vi "WLC Fitting_Final_v3_YCC.vi"(3 "initial parameters (Lp,Lc) or (Lc,K)":dbl[](array[numeric])=[40.0, 1750.0], 4 "Fitting Cluster":T1={"cr (um)"=0.0, "yr (V)"=0.0, "trap height(nm)"=300.0, "bead radius(nm)"=515.0, "Length offset"=550.0, "Upper Force(pN)"=500.0, "cr shift (nm)"=0.0, "yr shift (mV)"=0.0, "LaserPower (mW)"=4500.0, "conversion factor (V/um)"=0.0, "Stiffness (pN/nm)"=0.0, "xDNA cut outside"=3000.0, "Lower Force(pN)"=5.0, "c for zbd"=0.002} {"c for zbd" format="%_6g"}, 5 "Enum":T2(ring)=enum."direct fit (Lp,Lc,K)", 6 "Load Stage-QPD data":path, 7 "T=Fit U or twoside\nF=Fit F":bool=TRUE, 8 "F+U data?":bool=TRUE, 9 "Finish Fitting":bool, 10 "Ready to Fit":bool, 11 "DataRecord type":enum32{"OneDirectionOnly?", "TwoSide Data"}(tab)) -> (0 "best fit parameters":dbl[](array[numeric]), 1 "r^2":dbl)   [LabVIEW 2014]
uses:
  SubVI/WLC-Fitting Cluster.ctl
  <vilib>/Utility/file.llb/Read From Spreadsheet File (DBL).vi
  <vilib>/gmath/NumericalOptimization/Nonlinear Curve Fit LM formula string.vi
  <vilib>/Utility/file.llb/Write To Spreadsheet File (DBL).vi
  <vilib>/gmath/NI_Gmath.lvlib
panel:
  out "error out":errorcluster
  in  "Given Lp (nm)":dbl=5.0
  in  "Lower Force (pN)":dbl=6.0
  in  "Upper Force (pN)":dbl=45.0
  in  "Set lower foce offset?":bool
  out "U-Force or twoside 2":dbl[](array[numeric])
  out "U-xDNA or twoside 2":dbl[](array[numeric])
  in  "initial guess K (pN)":dbl=1200.0
  out "OneDirectionOnly?":bool=TRUE
  in  "Fit \"+\"(RHS) ?":bool=TRUE
  in  "Fit One Side?":bool
  in  "Reverse sign?":bool=TRUE
  out "Cut-Force for eWLC (pN)":dbl[](array[numeric])
  out "best nonlinear fit extension (eWLC)":dbl[](array[numeric])
  in  "T=use stuckbead 7th order\nF=use slope 1st order calibrate":bool
  out "Force to be saved":dbl[](array[numeric])
  out "xDNA to be saved":dbl[](array[numeric])
  out "F-Force":dbl[](array[numeric])
  out "F-xDNA":dbl[](array[numeric])
  in  "F-yr shift (mV)":dbl
  in  "F-cr shift (nm)":dbl
  out "F-QPD signal (V)":dbl[](array[numeric])
  out "F-Stage Positions (um)":dbl[](array[numeric])
  in  "stuckbead path (dialog if empty)":path=path "D:/Calibration-Stuckbead-Scan/20181220/2/202224-x-Stuckbead Scan-6000.00-step 5.00 nm-QPD height 3.340-h0.txt"
  out "Save to Path":path
  out "best nonlinear fit force (M-S)":dbl[](array[numeric])
  in  "SaveName":enum16{"ForecExtension Only", "WLC Fitting"}(ring)
  in  "Save Calibrated Data?":bool
  out "U-Force or twoside":dbl[](array[numeric])
  out "U-xDNA or twoside":dbl[](array[numeric])
  out "Fitting Cluster for indicator":T1={"cr (um)"=0.0, "yr (V)"=0.0, "trap height(nm)"=0.0, "bead radius(nm)"=520.0, "Length offset"=0.0, "Upper Force(pN)"=0.0, "cr shift (nm)"=0.0, "yr shift (mV)"=0.0, "LaserPower (mW)"=0.0, "conversion factor (V/um)"=0.0, "Stiffness (pN/nm)"=0.0154, "xDNA cut outside"=0.0, "Lower Force(pN)"=5.0, "c for zbd"=0.0}
  in  "Tab Control":T3(tab)
  out "Stage-QPD Graph":T4(graph)
  out "U-Extension-Force Graph":cluster{"xDNA":dbl[], "Force":dbl[]}(graph)
  out "F-Extension-Force Graph":cluster{"xDNA":dbl[], "Force":dbl[]}(graph)
  out "All-Extension-Force Graph":T5(graph)
  out "Extension-Force and WLC Graph":cluster{"xDNA":dbl[], "Force":dbl[]}[](graph)
  out "All Extension-Force and WLC Graph":T6(graph)
  in  "Delete Outside Signal?":bool
  out "U-QPD signal or All QPD  (V)":dbl[](array[numeric])
  out "U-Stage Positions or All stage positions (um)":dbl[](array[numeric])
  out "Read-Extension (nm)":dbl[](array[numeric])
  out "Read-Force (pN)":dbl[](array[numeric])
  in  "T=Read QPD-Stage data\nF=Read Force-Extension data":bool=TRUE
  # "5180bp=1750.8 nm\n3281bp=1109.0 nm"
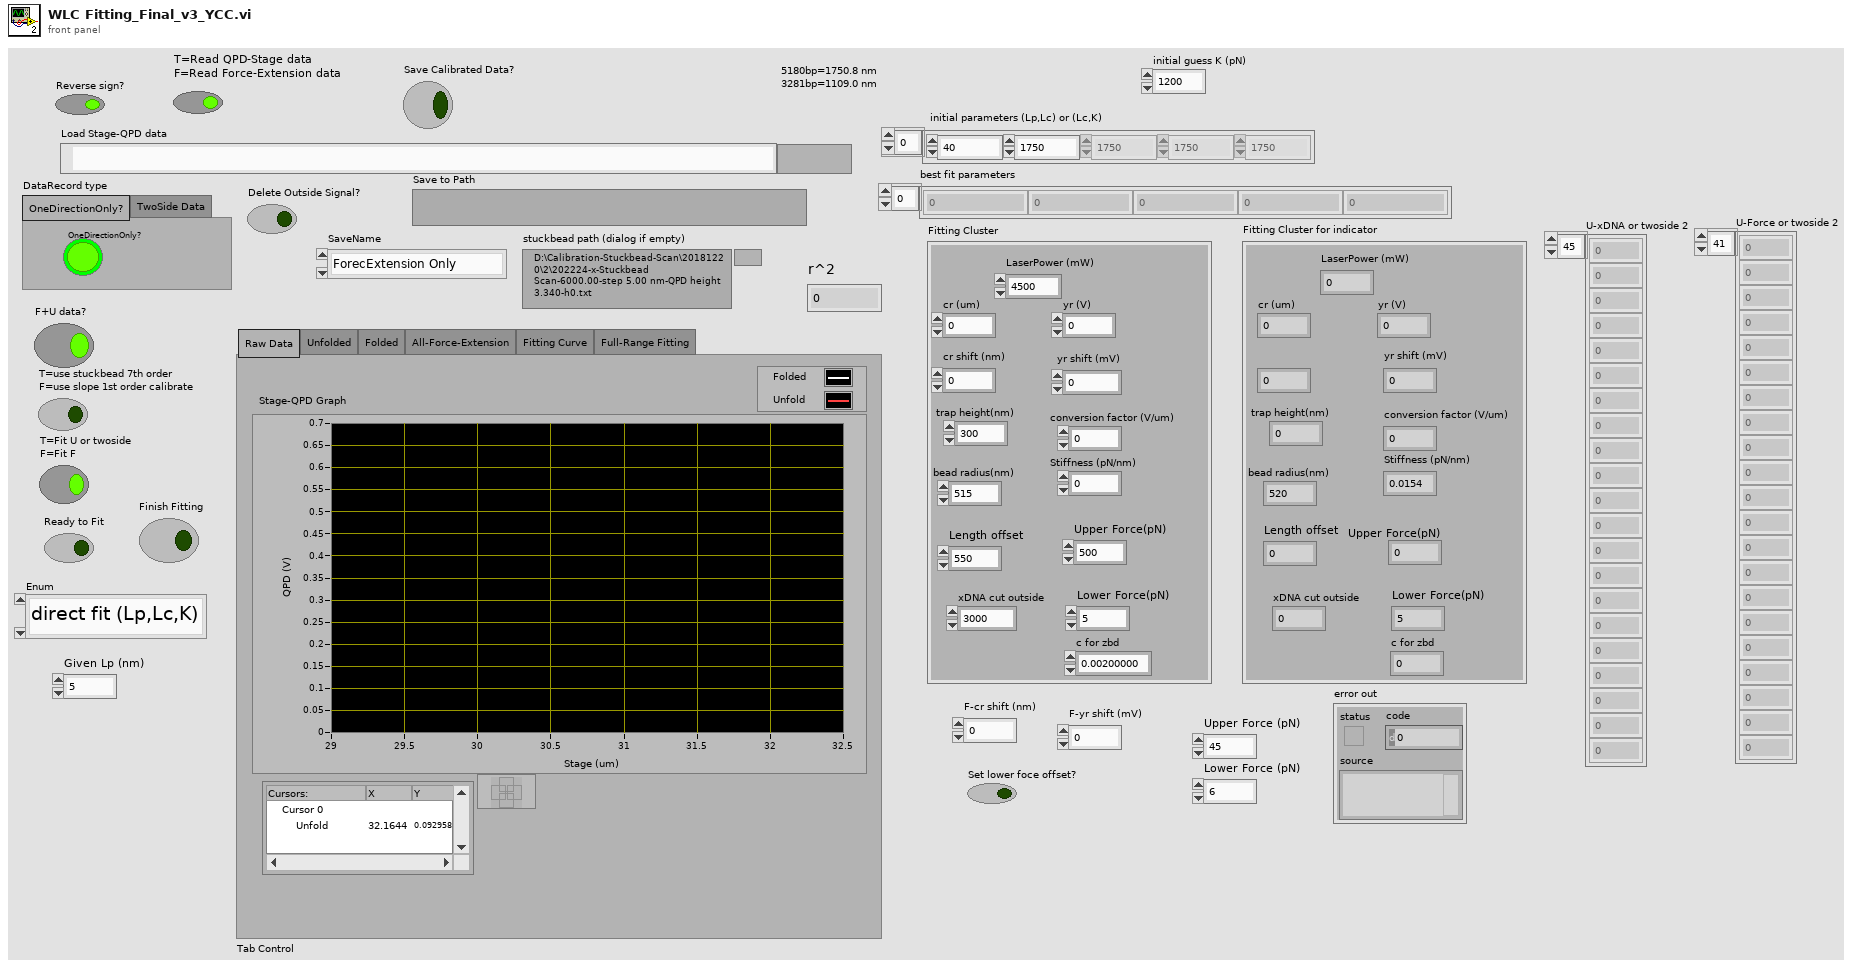
[diagram p1: front panel]
types:
  T1 = typedef "WLC-Fitting Cluster.ctl" = cluster{"cr (um)":dbl, "yr (V)":dbl, "trap height(nm)":dbl, "bead radius(nm)":dbl, "Length offset":dbl, "Upper Force(pN)":dbl, "cr shift (nm)":dbl, "yr shift (mV)":dbl, "LaserPower (mW)":dbl, "conversion factor (V/um)":dbl, "Stiffness (pN/nm)":dbl, "xDNA cut outside":dbl, "Lower Force(pN)":dbl, "c for zbd":dbl}
  T2 = enum16{" Marko-Siggia for centering", "Marko-Siggia", "direct fit (Lp,Lc,K)", "fit K (Lp,Lc,K)", "eWLC (Lp=45,Lc,K)"}
  T3 = enum32{"Raw Data", "Unfolded", "Folded", "All-Force-Extension", "Fitting Curve", "Full-Range Fitting"}
  T4 = cluster{"Sorted Stage Position (um)":dbl[], "Sorted QPD (V)":dbl[]}[]
  T5 = cluster{"Folded-xDNA":dbl[], "Folded-Force":dbl[]}[]
  T6 = cluster{"cut-full xDNA":dbl[], "cut-full Force":dbl[]}[]
  T7 = cluster{"model":string, "Parameters":string[], "x":string}
  T8 = cluster{"F-Stage Positions (um) ":dbl[], "F-QPD signal (V) ":dbl[]}
  T9 = cluster{"U-Stage Positions or All stage positions (um)":dbl[], "U-QPD signal or All QPD  (V)":dbl[]}
  T10 = cluster{"U-Stage Positions or All stage positions (um)":dbl[], "U-QPD signal or All QPD  (V)":dbl[]}[]
  T11 = cluster{"Folded-xDNA":dbl[], "Folded-xDNA":dbl[]}
  T12 = cluster{"cut-full xDNA":dbl[], "best nonlinear fit":dbl[]}
  T13 = cluster{"best nonlinear fit":dbl[], "cut-full Force":dbl[]}
  T14 = cluster{"cut-full xDNA":dbl[], "cut-full Force":dbl[]}
  T15 = cluster{"Fit Extension (nm)":dbl[], "Fit Force (pN)":dbl[]}
  T16 = cluster{"xDNA to be saved":dbl[], "Force to be saved":dbl[]}
  T17 = cluster{"xDNA to be saved":dbl[], "Force to be saved":dbl[]}[]
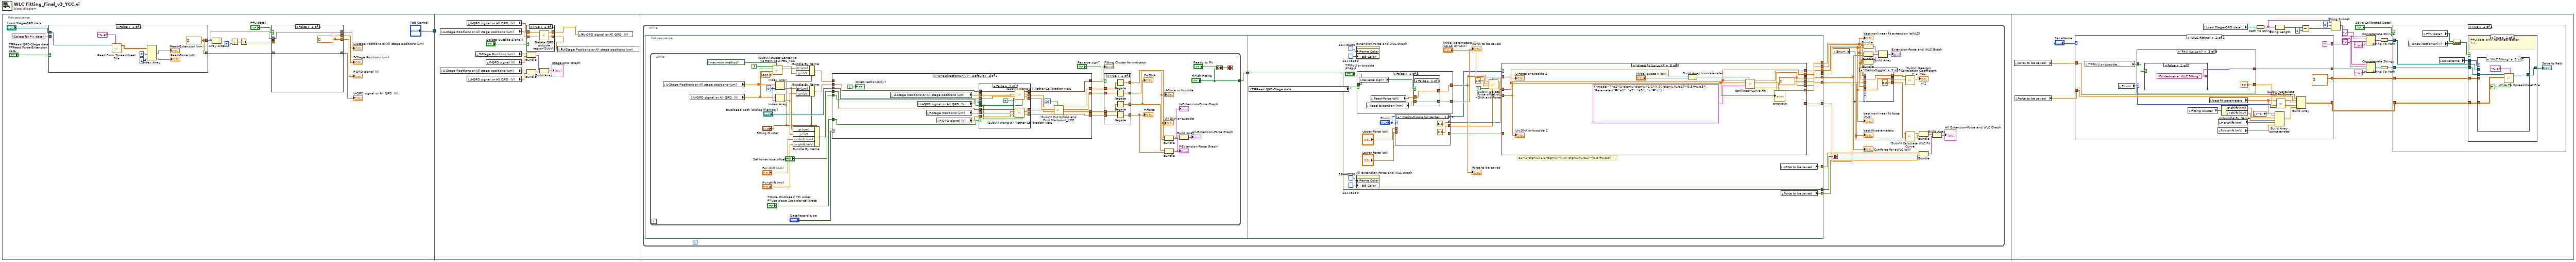
[diagram p0: block diagram]
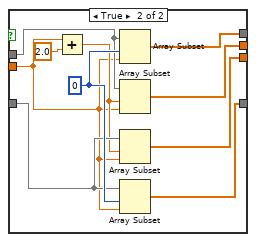
[diagram p2: hidden frame]
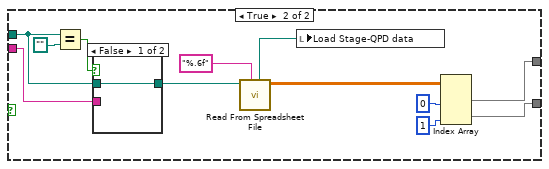
[diagram p3: hidden frame]
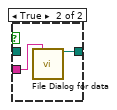
[diagram p4: hidden frame]
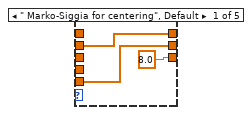
[diagram p6: hidden frame]
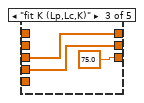
[diagram p7: hidden frame]
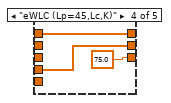
[diagram p8: hidden frame]
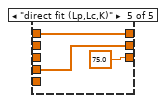
[diagram p9: hidden frame]
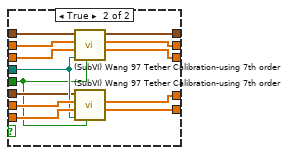
[diagram p11: hidden frame]
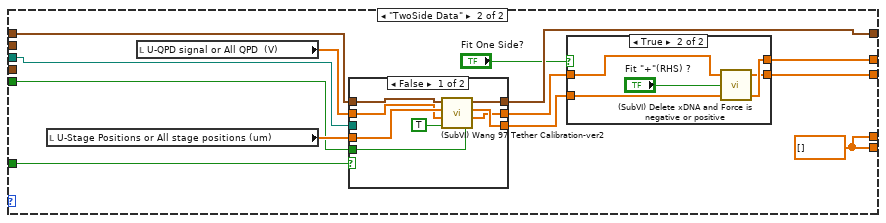
[diagram p12: hidden frame]
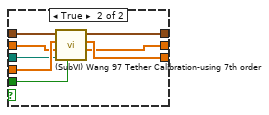
[diagram p14: hidden frame]
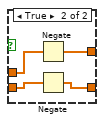
[diagram p15: hidden frame]
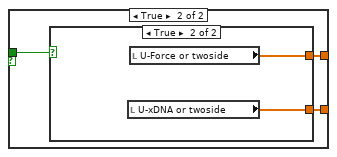
[diagram p16: hidden frame]
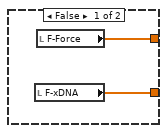
[diagram p17: hidden frame]
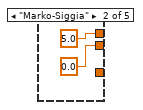
[diagram p18: hidden frame]
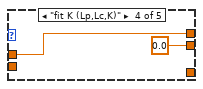
[diagram p20: hidden frame]
diagram:
  n1 = flat-sequence {
    tunnel: ["Tab Control"] -> w1
    tunnel: w1 -> [_]
    frame #0 {
      n2 = case shown="False" "T=Read QPD-Stage data\nF=Read Force-Extension data" {
        tunnel: [w35 w45] -> w11
        tunnel: [w35 w46] -> w6
        tunnel: "Select for F-x data" ("default name") -> [_ w42]
        tunnel: "Load Stage-QPD data" -> [w37 w39]
        frame False {
          w35 = dbl[] [] ("all rows")
          n3 = call-poly <vilib>:"Read From Spreadsheet File.vi"("format (%.3f)"="%.6f", "file path (dialog if empty)"=w37) -> ("all rows"=w32:dbl[][])  [unwired: 5 in, 4 out]
          n4 = Index Array(array=w32, index (col) #1=0 ("disabled index (col)"), index (col) #2=1 ("index (col)")) -> (element #1=→"Read-Extension (nm)":dbl[], element #2=→"Read-Force (pN)":dbl[])  [unwired: 2 in]
        }
        frame True {
          n5 = Equal?(x=w39, y=path "") -> (x = y?=w40:bool)
          n6 = case shown="False" w40 {
            tunnel: [w50 w51] -> w43
            tunnel: w42 -> [_ w52]
            tunnel: w39 -> [w50 _]
            frame False {
            }
            frame True {
              n7 = call "File Dialog for data"("prompt"=w52) -> ("selected path"=w51:path)  [unwired: 11 in, 3 out]
            }
          }
          n8 = call-poly <vilib>:"Read From Spreadsheet File.vi"("format (%.3f)"="%.6f", "file path (dialog if empty)"=w43) -> ("all rows"=w49:dbl[][], "new file path (Not A Path if cancelled)"=w38:path)  [unwired: 5 in, 3 out]
          n9 = local write "Load Stage-QPD data"(w38) -> ()
          n10 = Index Array(array=w49, index (col) #1=0 ("disabled index (col)"), index (col) #2=1 ("index (col)")) -> (element #1=w46:dbl[], element #2=w45:dbl[])  [unwired: 2 in]
        }
      }
      n11 = Array Size(array=w6) -> (size(s)=w7:i32)
      n12 = Divide(x=w7, y=2) -> (x/y=w5:dbl)
      n13 = Decrement(x=w5) -> (x-1=w4:dbl)
      n14 = case shown="False" "F+U data?" {
        tunnel: w6 -> [w19 w25]
        tunnel: w11 -> [w18 w26]
        tunnel: [w19 w29] -> w10
        tunnel: [w18 w27] -> w9
        tunnel: w4 -> [_ w20]
        tunnel: [w17 w24] -> w3
        tunnel: [w17 w23] -> w2
        frame False {
          w17 = dbl[] []
        }
        frame True {
          w28 = 0 ("index")
          n15 = Add(x=w20, y=2.0) -> (x+y=w21:dbl)
          n16 = Array Subset(array=w25, index=w28, length=w20) -> (w29:dbl[])
          n17 = Array Subset(array=w25, index=w21, length=w20) -> (w24:dbl[])
          n18 = Array Subset(array=w26, index=w21, length=w20) -> (w23:dbl[])
          n19 = Array Subset(array=w26, index=w28, length=w20) -> (w27:dbl[])
        }
      }
      "U-Stage Positions or All stage positions (um)" <- w10
      "U-QPD signal or All QPD  (V)" <- w9
      "F-Stage Positions (um)" <- w3
      "F-QPD signal (V)" <- w2
    }
    frame #1 {
      n20 = local read "U-Stage Positions or All stage positions (um)"() -> (w63:dbl[])
      n21 = local read "U-Stage Positions or All stage positions (um)"() -> (w61:dbl[])
      n22 = local read "U-QPD signal or All QPD  (V)"() -> (w62:dbl[])
      n23 = local read "U-QPD signal or All QPD  (V)"() -> (w60:dbl[])
      n24 = local read "F-Stage Positions (um)"() -> (w56:dbl[])
      n25 = local read "F-QPD signal (V)"() -> (w55:dbl[])
      n26 = case shown="True" "Delete Outside Signal?" {
        tunnel: w62 -> [w66 w70]
        tunnel: w63 -> [w65 w69]
        tunnel: [w66 w68] -> w53
        tunnel: [w65 w67] -> w54
        frame False {
        }
        frame True {
          n27 = call "Delete QPD outside region(SubVI).vi"("Position Array In"=w69, "QPD signal In"=w70) -> ("Position Array Out"=w67:dbl[], "QPD signal Out"=w68:dbl[])  [unwired: 8 in]
        }
      }
      n28 = Bundle("F-Stage Positions (um)"=w56, "F-QPD signal (V)"=w55) -> (w59:T8)  [unwired: 1 in]
      n29 = Bundle("U-Stage Positions or All stage positions (um)"=w61, "U-QPD signal or All QPD  (V)"=w60) -> (w58:T9)  [unwired: 1 in]
      n30 = Build Array(w59, w58) -> (→"Stage-QPD Graph":T10)
      n31 = local write "U-Stage Positions or All stage positions (um)"(w54) -> ()
      n32 = local write "U-QPD signal or All QPD  (V)"(w53) -> ()
    }
    frame #2 {
      n33 = while {
        stop <- w85 stop-if-true
        n34 = flat-sequence {
          tunnel: [w111] -> w86
          tunnel: [w269] -> w91
          tunnel: [w268] -> w82
          tunnel: [w266] -> w88
          tunnel: [w265] -> w92
          tunnel: [w264] -> w87
          tunnel: [w263] -> w94
          tunnel: [w262] -> w85
          tunnel: w86 -> [w262]
          tunnel: [w249] -> w83
          tunnel: [w248] -> w74
          tunnel: [w247] -> w73
          frame #0 {
            n35 = while {
              tunnel: ["Finish Fitting"] -> w111
              stop <- w115 stop-if-true
              w147 = 0 ("index")
              n36 = local read "U-Stage Positions or All stage positions (um)"() -> (w136:dbl[])
              n37 = local read "U-QPD signal or All QPD  (V)"() -> (w135:dbl[])
              n38 = call "(SubVI) Guess Center xc yc From Raw FEC_YCC.vi"("Enum"=enum16{"parity method", "max-min method"}."max-min method", "avg range for QPD center (nm)"=600.0, "QPD array (V)"=w135, "Stage array(um)"=w136, "Read data?"=FALSE) -> ("Guess-QPD-center (V)"=w133:dbl, "Guess-stage-center(um)"=w134:dbl)  [unwired: 1 in, 2 out]
              n39 = Index Array(array=w136, index=w147) -> (element=w144:dbl)
              n40 = Index Array(array=w135, index=w147) -> (element=w143:dbl)
              n41 = Bundle By Name(cluster="Fitting Cluster", "cr (um)"=w144, "yr (V)"=w143, "cr shift (nm)"="F-cr shift (nm)", "yr shift (mV)"="F-yr shift (mV)") -> (w140:T1)
              n42 = Bundle By Name(cluster="Fitting Cluster", "cr (um)"=w134, "yr (V)"=w133) -> (w132:T1)
              n43 = Bundle By Name(cluster="Fitting Cluster", "cr (um)"=w144, "yr (V)"=w143) -> (w146:T1)
              n44 = case shown="\"OneDirectionOnly?\", Default" "DataRecord type" {
                tunnel: w146 -> [w177 _]
                tunnel: [w178 w215] -> w145
                tunnel: w140 -> [w173 _]
                tunnel: w132 -> [_ w218]
                tunnel: [w167 w208] -> w129
                tunnel: [w166 w207] -> w123
                tunnel: [w165 w214] -> w128
                tunnel: [w164 w214] -> w127
                tunnel: "T=use stuckbead 7th order\nF=use slope 1st order calibrate" -> [w163 w213]
                tunnel: "stuckbead path (dialog if empty)" -> [w162 w212]
                tunnel: "Set lower foce offset?" -> [w160 w206]
                frame "OneDirectionOnly?", Default {
                  n45 = local read "U-Stage Positions or All stage positions (um)"() -> (w176:dbl[])
                  n46 = local read "U-QPD signal or All QPD  (V)"() -> (w179:dbl[])
                  n47 = local read "F-Stage Positions (um)"() -> (w175:dbl[])
                  n48 = local read "F-QPD signal (V)"() -> (w174:dbl[])
                  n49 = case shown="False" w163 {
                    tunnel: w179 -> [w191 w205]
                    tunnel: [w190 w204] -> w178
                    tunnel: w177 -> [w182 w203]
                    tunnel: w176 -> [w192 w202]
                    tunnel: w175 -> [w188 w201]
                    tunnel: w174 -> [w187 w200]
                    tunnel: w162 -> [_ w199]
                    tunnel: w173 -> [w189 w198]
                    tunnel: [w186 w197] -> w171
                    tunnel: [w185 w196] -> w170
                    tunnel: [w184 w195] -> w169
                    tunnel: [w183 w194] -> w168
                    tunnel: w160 -> [w180 w193]
                    frame False {
                      w181 = TRUE ("X=T\nY=F")
                      n50 = call "(SubVI) Wang 97 Tether Calibration-ver2.vi"("Set lower foce offset?"=w180, "X=T\nY=F"=w181, "QPD signal"=w191, "Stage Position"=w192, "Fitting Cluster"=w182) -> ("Force"=w185:dbl[], "xDNA"=w186:dbl[], "output cluster"=w190:T1)
                      n51 = call "(SubVI) Wang 97 Tether Calibration-ver2.vi"("Set lower foce offset?"=w180, "X=T\nY=F"=w181, "QPD signal"=w187, "Stage Position"=w188, "Fitting Cluster"=w189) -> ("Force"=w183:dbl[], "xDNA"=w184:dbl[])  [unwired: 1 out]
                    }
                    frame True {
                      n52 = call "(SubVI) Wang 97 Tether Calibration-using 7th order.vi"("Set lower foce offset?"=w193, "stuckbead path (dialog if empty)"=w199, "QPD signal"=w205, "Stage Position"=w202, "Fitting Cluster"=w203) -> ("Force"=w196:dbl[], "xDNA"=w197:dbl[], "output cluster"=w204:T1)  [unwired: 2 in, 2 out]
                      n53 = call "(SubVI) Wang 97 Tether Calibration-using 7th order.vi"("Set lower foce offset?"=w193, "stuckbead path (dialog if empty)"=w199, "QPD signal"=w200, "Stage Position"=w201, "Fitting Cluster"=w198) -> ("Force"=w194:dbl[], "xDNA"=w195:dbl[])  [unwired: 2 in, 3 out]
                    }
                  }
                  n54 = call "(SubVI) Cut Unfold and Fold Startpoint_YCC.vi"("number to cut"=10, "Folded-Force in"=w168, "Folded-xDNA in"=w169, "Unfolded-Force"=w170, "Unfolded-xDNA"=w171) -> ("Folded-Force"=w164:dbl[], "Folded-xDNA"=w165:dbl[], "Unfolded-Force"=w166:dbl[], "Unfolded-xDNA"=w167:dbl[])  [unwired: 3 in]
                  "OneDirectionOnly?" <- TRUE
                }
                frame "TwoSide Data" {
                  w214 = dbl[] [] ("Folded-xDNA")
                  n55 = local read "U-Stage Positions or All stage positions (um)"() -> (w217:dbl[])
                  n56 = local read "U-QPD signal or All QPD  (V)"() -> (w216:dbl[])
                  n57 = case shown="False" w213 {
                    tunnel: w218 -> [w233 w241]
                    tunnel: w217 -> [w232 w240]
                    tunnel: w216 -> [w231 w239]
                    tunnel: [w230 w237] -> w215
                    tunnel: [w229 w236] -> w209
                    tunnel: [w228 w235] -> w210
                    tunnel: w212 -> [_ w238]
                    tunnel: w206 -> [w226 w234]
                    frame False {
                      n58 = call "(SubVI) Wang 97 Tether Calibration-ver2.vi"("Set lower foce offset?"=w226, "X=T\nY=F"=TRUE ("X=T\nY=F"), "QPD signal"=w231, "Stage Position"=w232, "Fitting Cluster"=w233) -> ("Force"=w228:dbl[], "xDNA"=w229:dbl[], "output cluster"=w230:T1)
                    }
                    frame True {
                      n59 = call "(SubVI) Wang 97 Tether Calibration-using 7th order.vi"("Set lower foce offset?"=w234, "stuckbead path (dialog if empty)"=w238, "QPD signal"=w239, "Stage Position"=w240, "Fitting Cluster"=w241) -> ("Force"=w235:dbl[], "xDNA"=w236:dbl[], "output cluster"=w237:T1)  [unwired: 2 in, 2 out]
                    }
                  }
                  n60 = case shown="True" "Fit One Side?" {
                    tunnel: w210 -> [w220 w224]
                    tunnel: w209 -> [w219 w223]
                    tunnel: [w219 w222] -> w208
                    tunnel: [w220 w221] -> w207
                    frame False {
                    }
                    frame True {
                      n61 = call "(SubVI) Delete xDNA and Force is negative or positive.vi"("xDNA"=w223, "T=positive (RHS)\nF=negative (LHS)"="Fit \"+\"(RHS) ?", "Force"=w224) -> ("xDNA-cut"=w222:dbl[], "Force-cut"=w221:dbl[])  [unwired: 1 in]
                    }
                  }
                }
              }
              "Fitting Cluster for indicator" <- w145
              n62 = case shown="True" "Reverse sign?" {
                tunnel: w129 -> [w151 w153]
                tunnel: w128 -> [w149 w159]
                tunnel: w127 -> [w148 w158]
                tunnel: [w148 w157] -> w126
                tunnel: [w149 w156] -> w125
                tunnel: [w151 w152] -> w124
                tunnel: w123 -> [w150 w155]
                tunnel: [w150 w154] -> w122
                frame False {
                }
                frame True {
                  n63 = Negate(x=w153) -> (-x=w152:dbl[])
                  n64 = Negate(x=w155) -> (-x=w154:dbl[])
                  n65 = Negate(x=w159) -> (-x=w156:dbl[])
                  n66 = Negate(x=w158) -> (-x=w157:dbl[])
                }
              }
              "U-xDNA or twoside" <- w124
              "U-Force or twoside" <- w122
              "F-xDNA" <- w125
              "F-Force" <- w126
              n67 = Bundle("xDNA-cut"=w124, "Force-cut"=w122) -> (w137:cluster{"xDNA-cut":dbl[], "Force-cut":dbl[]})  [unwired: 1 in]
              "U-Extension-Force Graph" <- w137
              n68 = Bundle("Folded-xDNA"=w125, "Folded-xDNA"=w126) -> (w138:T11)  [unwired: 1 in]
              "F-Extension-Force Graph" <- w138
              n69 = Build Array(w138, w137) -> (→"All-Extension-Force Graph":cluster{"xDNA-cut":dbl[], "Force-cut":dbl[]}[])
              n70 = Or(x="Ready to Fit", y="Finish Fitting") -> (x .or. y?=w115:bool)
            }
          }
          frame #1 {
            # "a2*(1*sign(u)-1/2*sign(u)*(4.07/sign(u)/u/a1)**(0.5)+u/a3);"
            n71 = local read "T=Read QPD-Stage data\nF=Read Force-Extension data"() -> (w242:bool)
            n72 = property on="Extension-Force and WLC Graph" class="XYGraph (strict)"("Frame Color"=u32 16448250, "BG Color"=u32 16448250) -> ()  [unwired: 2 in, 2 out]
            n73 = property on="All Extension-Force and WLC Graph" class="XYGraph (strict)"("Frame Color"=u32 16448250, "BG Color"=u32 16448250) -> ()  [unwired: 2 in, 2 out]
            n74 = case shown="False" w242 {
              tunnel: "T=Fit U or twoside\nF=Fit F" -> [_ w284]
              tunnel: [w271 w283] -> w257
              tunnel: [w272 w282] -> w256
              frame False {
                n75 = local read "Reverse sign?"() -> (w275:bool)
                n76 = local read "Read-Extension (nm)"() -> (w273:dbl[])
                n77 = local read "Read-Force (pN)"() -> (w274:dbl[])
                n78 = case shown="False" w275 {
                  tunnel: w274 -> [w277 w281]
                  tunnel: w273 -> [w276 w279]
                  tunnel: [w277 w280] -> w272
                  tunnel: [w276 w278] -> w271
                  frame False {
                  }
                  frame True {
                    n79 = Negate(x=w281) -> (-x=w280:dbl[])
                    n80 = Negate(x=w279) -> (-x=w278:dbl[])
                  }
                }
              }
              frame True {
                n81 = case shown="True" w284 {
                  tunnel: [w286 w288] -> w283
                  tunnel: [w285 w287] -> w282
                  frame False {
                    n82 = local read "F-xDNA"() -> (w286:dbl[])
                    n83 = local read "F-Force"() -> (w285:dbl[])
                  }
                  frame True {
                    n84 = local read "U-xDNA or twoside"() -> (w288:dbl[])
                    n85 = local read "U-Force or twoside"() -> (w287:dbl[])
                  }
                }
              }
            }
            "xDNA to be saved" <- w257
            "Force to be saved" <- w256
            n86 = case shown="\" Marko-Siggia for centering\", Default" "Enum" {
              tunnel: [0.0 0.0 w293 0.0 ("Lower Force (pN)") w298] -> w254
              tunnel: [5.0 5.0 w294 w295 w299] -> w253
              tunnel: "Upper Force (pN)" -> [_ _ w294 w295 w299]
              tunnel: "Lower Force (pN)" -> [_ _ w293 _ w298]
              tunnel: [_ _ _ _ "Given Lp (nm)"] -> w250
              frame " Marko-Siggia for centering", Default {
              }
              frame "Marko-Siggia" {
              }
              frame "direct fit (Lp,Lc,K)" {
              }
              frame "fit K (Lp,Lc,K)" {
              }
              frame "eWLC (Lp=45,Lc,K)" {
              }
            }
            n87 = call "(SubVI) Delete Force offset of xDNA and Force.vi"("Force"=w256, "Upper Force (pN)"=w253, "xDNA"=w257, "force constant"=1.0, "Lower Force (pN)"=w254, "Set lower foce offset?"=TRUE) -> ("cut-full Force"=w258:dbl[], "cut-full xDNA"=w259:dbl[])  [unwired: 1 in]
            n88 = case shown="\"direct fit (Lp,Lc,K)\"" "Enum" {
              tunnel: "initial parameters (Lp,Lc) or (Lc,K)" -> [w306 w313 w330 w331 w351]
              tunnel: w258 -> [w300 w311 w326 w342 w345]
              tunnel: w259 -> [w301 w310 w327 w334 w347]
              tunnel: [w304 w315 dbl[] [] ("best nonlinear fit") dbl[] [] ("best nonlinear fit") dbl[] [] ("best nonlinear fit")] -> w269
              tunnel: [w305 w314 w324 w332 w349] -> w268
              tunnel: [w301 w310 w327 w334 w347] -> w266
              tunnel: [w300 w311 w326 w342 w345] -> w265
              tunnel: [dbl[] [] ("best nonlinear fit extension for eWLC") w312 w329 w340 w348] -> w264
              tunnel: [dbl[] [] ("Cut-Force (pN)") w312 w326 w338 w345] -> w263
              tunnel: w250 -> [_ _ w317 _ _]
              tunnel: [_ _ _ w333 _] -> w249
              frame " Marko-Siggia for centering", Default {
                n89 = Build Array (concatenate)(w306, dbl[] [0.1, 0.1] ("element")) -> (w307:dbl[])
                n90 = call-poly <vilib>:"Nonlinear Curve Fit.vi"("Y"=w300, "initial parameters"=w307, "X"=w301, "model description"=T7 {"model"="4.08687*(1/a1)*(sign(u-a3)*1/4*(1-sign(u-a3)*(u-a3)/a2)^(-2)-(1/4*sign(u-a3))+(u-a3)/a2)+a4", "Parameters"=["a1", "a2", "a3", "a4"], "x"="u"}) -> ("best nonlinear fit"=w304:dbl[], "best fit parameters"=w305:dbl[])  [unwired: 3 in, 7 out]
              }
              frame "Marko-Siggia" {
                w312 = dbl[] [] ("best nonlinear fit extension for eWLC")
                n91 = call-poly <vilib>:"Nonlinear Curve Fit.vi"("Y"=w311, "initial parameters"=w313, "X"=w310, "model description"=T7 {"model"="4.08687*(1/a1)*(sign(u)*1/4*(1-sign(u)*u/a2)^(-2)-(1/4*sign(u))+u/a2)", "Parameters"=["a1", "a2"], "x"="u"}) -> ("best nonlinear fit"=w315:dbl[], "best fit parameters"=w314:dbl[])  [unwired: 3 in, 7 out]
              }
              frame "eWLC (Lp=45,Lc,K)" {
                n92 = Number To Decimal String(number=w317) -> (decimal integer string=w323:string)  [unwired: 1 in]
                n93 = Concatenate Strings("a1*(1*sign(u)-sign(u)*1/2*(4.07/sign(u)/u/" ("model"), w323, ")^(0.5)+u/a2)" ("model")) -> (w319:string)
                n94 = Bundle(cluster=T7 {"model"="a1*(1*sign(u)-sign(u)*1/2*(4.07/sign(u)/u/45)^(0.5)+u/a2)", "Parameters"=["a1", "a2"], "x"="u"} ("model description"), "model"=w319) -> (w318:T7)  [unwired: 2 in]
                n95 = call-poly <vilib>:"Nonlinear Curve Fit.vi"("Y"=w327, "initial parameters"=w330, "X"=w326, "model description"=w318) -> ("best nonlinear fit"=w329:dbl[], "best fit parameters"=w325:dbl[])  [unwired: 3 in, 7 out]
                n96 = Build Array (concatenate)(w317, w325) -> (w324:dbl[])
              }
              frame "fit K (Lp,Lc,K)" {
                n97 = call "Serial fit Lc and K.vi"("Extension (nm)"=w334, "Force (pN)"=w342, "initial parameters for WLC (Lp,Lc)"=w331) -> ("Cut-Extenison (nm)"=w333:dbl[], "Cut-Force (pN)"=w338:dbl[], "best fit parameters for eWLC (Lp,Lc,K)"=w332:dbl[], "best fit parameters for WLC"=w341:dbl[], "best nonlinear fit extension for eWLC"=w340:dbl[])  [unwired: 1 in]
                n98 = Delete From Array(array=w332, length=1, index=0) -> (array with subset deleted=w335:dbl[])  [unwired: 1 out]
                n99 = Build Array (concatenate)(w341, w335) -> ()  [unwired: 1 out]
              }
              frame "direct fit (Lp,Lc,K)" {
                n100 = Build Array (concatenate)(w351, "initial guess K (pN)") -> (w350:dbl[])
                n101 = call-poly <vilib>:"Nonlinear Curve Fit.vi"("Y"=w347, "initial parameters"=w350, "X"=w345, "model description"=T7 {"model"="a2*(1*sign(u)-sign(u)*1/2*(4.07/sign(u)/u/a1)^(0.5)+u/a3)", "Parameters"=["a1", "a2", "a3"], "x"="u"}) -> ("best nonlinear fit"=w348:dbl[], "best fit parameters"=w349:dbl[], "error out"=→"error out":errorcluster)  [unwired: 3 in, 6 out]
                "U-xDNA or twoside 2" <- w347
                "U-Force or twoside 2" <- w345
              }
            }
            n102 = local read "xDNA to be saved"() -> (w248:dbl[])
            n103 = local read "Force to be saved"() -> (w247:dbl[])
          }
        }
        n104 = local read "Enum"() -> (w81:T2)
        n105 = Bundle("cut-full xDNA"=w88, "best nonlinear fit"=w91) -> (w95:T12)  [unwired: 1 in]
        n106 = Bundle("best nonlinear fit"=w87, "cut-full Force"=w94) -> (w84:T13)  [unwired: 1 in]
        n107 = Bundle("cut-full xDNA"=w88, "cut-full Force"=w92) -> (w78:T14)  [unwired: 1 in]
        n108 = case shown="\"Marko-Siggia\"" w81 {
          tunnel: w92 -> [w98 w101 _ _ _]
          tunnel: w91 -> [w97 w100 _ _ _]
          tunnel: [w98 w101 w103 w107 w109] -> w90
          tunnel: [w97 w100 w104 w106 w110] -> w89
          tunnel: w88 -> [_ _ _ w107 w109]
          tunnel: w87 -> [_ _ w104 w106 w110]
          tunnel: w83 -> [_ _ w103 _ _]
          tunnel: [8.0 ("Force Upper Limit") 8.0 ("Force Upper Limit") 75.0 ("Force Upper Limit") 75.0 ("Force Upper Limit") 75.0 ("Force Upper Limit")] -> w71
          frame " Marko-Siggia for centering", Default {
          }
          frame "Marko-Siggia" {
          }
          frame "fit K (Lp,Lc,K)" {
          }
          frame "eWLC (Lp=45,Lc,K)" {
          }
          frame "direct fit (Lp,Lc,K)" {
          }
        }
        n109 = Build Array(w95, w84, w78) -> (→"Extension-Force and WLC Graph":T6)
        n110 = call "(SubVI) Pearson Correlation Coefficient r^2_YCC.vi"("best fit Data"=w89, "Data"=w90) -> ("r^2"=→"r^2":dbl)  [unwired: 4 in, 1 out]
        n111 = call "(SubVI) Calculate WLC Fit Curve.vi"("Enum 2"=w81, "Force Upper Limit"=w71, "BestFit"=w82) -> ("Fit Force (pN)"=w79:dbl[], "Fit Extension (nm)"=w80:dbl[])  [unwired: 4 in]
        n112 = Bundle("Fit Extension (nm)"=w80, "Fit Force (pN)"=w79) -> (w77:T15)  [unwired: 1 in]
        n113 = Bundle("xDNA to be saved"=w74, "Force to be saved"=w73) -> (w72:T16)  [unwired: 1 in]
        n114 = Build Array(w77, w72) -> (→"All Extension-Force and WLC Graph":T17)
        "best nonlinear fit force (M-S)" <- w91
        "best fit parameters" <- w82
        "best nonlinear fit extension (eWLC)" <- w87
        "Cut-Force for eWLC (pN)" <- w94
      }
    }
    frame #3 {
      n115 = local read "xDNA to be saved"() -> (w354:dbl[])
      n116 = local read "Force to be saved"() -> (w353:dbl[])
      n117 = case shown="\"WLC Fitting\"" "SaveName" {
        tunnel: [w384 w404] -> w366
        tunnel: [w383 w420] -> w363
        tunnel: [w382 "" ("string")] -> w358
        tunnel: [w381 dbl[][] []] -> w355
        tunnel: w354 -> [w378 w417]
        tunnel: w353 -> [w377 w416]
        frame "ForecExtension Only", Default {
          n118 = local read "OneDirectionOnly?"() -> (w376:bool)
          n119 = local read "F+U data?"() -> (w380:bool)
          n120 = And(x=w380, y=w376) -> (x .and. y?=w379:bool)
          n121 = case shown="True" w379 {
            tunnel: [w391 "U-ForecExtension Only" ("string")] -> w384
            tunnel: [w388 w398] -> w383
            tunnel: ["" ("string") "F-ForecExtension Only" ("string")] -> w382
            tunnel: [dbl[][] [] w394] -> w381
            tunnel: w378 -> [w387 _]
            tunnel: w377 -> [w386 _]
            tunnel: w376 -> [w385 _]
            frame False {
              n122 = case shown="True" w385 {
                tunnel: ["twoside-ForecExtension Only" ("string") "U-ForecExtension Only" ("string")] -> w391
                frame False {
                }
                frame True {
                }
              }
              n123 = Build Array(w387, w386) -> (w388:dbl[][])
            }
            frame True {
              n124 = local read "U-xDNA or twoside"() -> (w400:dbl[])
              n125 = local read "U-Force or twoside"() -> (w399:dbl[])
              n126 = local read "F-xDNA"() -> (w397:dbl[])
              n127 = local read "F-Force"() -> (w396:dbl[])
              n128 = Build Array(w397, w396) -> (w394:dbl[][])
              n129 = Build Array(w400, w399) -> (w398:dbl[][])
            }
          }
        }
        frame "WLC Fitting" {
          n130 = local read "T=Fit U or twoside\nF=Fit F"() -> (w403:bool)
          n131 = local read "Enum"() -> (w413:T2)
          n132 = case shown="\"fit K (Lp,Lc,K)\"" w413 {
            tunnel: [90.0 ("Force Upper Limit") 90.0 ("Force Upper Limit") 90.0 ("Force Upper Limit") 150.0 ("Force Upper Limit") 90.0 ("Force Upper Limit")] -> w415
            tunnel: ["MS-WLC Fitting" ("string") w424 w429 w434 w439] -> w404
            tunnel: w403 -> [_ w423 w428 w433 w438]
            frame " Marko-Siggia for centering", Default {
            }
            frame "Marko-Siggia" {
              n133 = case shown="True" w423 {
                tunnel: ["Folded-MS-WLC Fitting" ("string") "Unfolded-MS-WLC Fitting" ("string")] -> w424
                frame False {
                }
                frame True {
                }
              }
            }
            frame "fit K (Lp,Lc,K)" {
              n134 = case shown="False" w428 {
                tunnel: ["Folded-serial WLC Fitting" ("string") "Unfolded-serial WLC Fitting" ("string")] -> w429
                frame False {
                }
                frame True {
                }
              }
            }
            frame "eWLC (Lp=45,Lc,K)" {
              n135 = case shown="True" w433 {
                tunnel: ["Folded-eWLC Fitting Lp45" ("string") "Unfolded-eWLC Fitting Lp45" ("string")] -> w434
                frame False {
                }
                frame True {
                }
              }
            }
            frame "direct fit (Lp,Lc,K)" {
              n136 = case shown="False" w438 {
                tunnel: ["Folded-eWLC Fitting" ("string") "Unfolded-eWLC Fitting" ("string")] -> w439
                frame False {
                }
                frame True {
                }
              }
            }
          }
          n137 = local read "Fitting Cluster"() -> (w409:T1)
          n138 = local read "best fit parameters"() -> (w412:dbl[])
          n139 = local read "F-yr shift (mV)"() -> (w405:dbl)
          n140 = local read "F-cr shift (nm)"() -> (w406:dbl)
          n141 = Unbundle By Name(w409) -> ("cr shift (nm)"=w408:dbl, "yr shift (mV)"=w407:dbl)
          n142 = local read "r^2"() -> (w411:dbl)
          n143 = Build Array (concatenate)(w412, w411, w408, w407, w406, w405) -> (w410:dbl[])
          n144 = call "(SubVI) Calculate WLC Fit Curve.vi"("Enum 2"=w413, "Force Upper Limit"=w415, "BestFit"=w412) -> ("Fit Force (pN)"=w414:dbl[], "Fit Extension (nm)"=w402:dbl[])  [unwired: 4 in]
          n145 = Build Array(w417, w416, w402, w414, w410) -> (w420:dbl[][])
        }
      }
      n146 = local read "Load Stage-QPD data"() -> (w375:path)
      n147 = Path To String(path=w375) -> (string=w373:string)
      n148 = String Length(string=w373) -> (length=w372:i32)
      n149 = Subtract(x=w372, y=4) -> (x-y=w369:i32)
      n150 = String Subset(string=w373, offset (0)=0, length (rest)=w369) -> (substring=w360:string)
      n151 = Concatenate Strings(w360, "-" ("string"), w358, ".txt" ("string")) -> (w361:string)
      n152 = Concatenate Strings(w360, "-" ("string"), w366, ".txt" ("string")) -> (w362:string)
      n153 = String To Path(string=w361) -> (path=w356:path)
      n154 = String To Path(string=w362) -> (path=w364:path)
      n155 = case shown="True" "Save Calibrated Data?" {
        tunnel: w364 -> [_ w451]
        tunnel: w363 -> [_ w450]
        tunnel: w356 -> [_ w449]
        tunnel: w355 -> [_ w448]
        frame False {
        }
        frame True {
          n156 = local read "OneDirectionOnly?"() -> (w446:bool)
          n157 = local read "F+U data?"() -> (w445:bool)
          n158 = local read "SaveName"() -> (w443:enum16{"ForecExtension Only", "WLC Fitting"})
          n159 = And(x=w445, y=w446) -> (x .and. y?=w444:bool)
          n160 = case shown="True" w444 {
            tunnel: w451 -> [w453 w462]
            tunnel: w450 -> [w454 w461]
            tunnel: w449 -> [_ w460]
            tunnel: w448 -> [_ w459]
            tunnel: [w452 w458] -> w447
            tunnel: w443 -> [_ w457]
            frame False {
              # "twoside data or Unfolded data only"
              n161 = call-poly <vilib>:"Write To Spreadsheet File.vi"("transpose? (no:F)"=TRUE, "format (%.3f)"="%.6f", "2D data"=w454, "file path (dialog if empty)"=w453) -> ("new file path (Not A Path if cancelled)"=w452:path)  [unwired: 4 in]
            }
            frame True {
              # "F+U data only for onedirection\nT,T"
              n162 = case shown="\"WLC Fitting\"" w457 {
                tunnel: w462 -> [w470 w472]
                tunnel: w461 -> [w469 w473]
                tunnel: w460 -> [w466 _]
                tunnel: w459 -> [w465 _]
                tunnel: [w463 w471] -> w458
                frame "ForecExtension Only", Default {
                  w467 = "%.6f" ("format (%.3f)")
                  n163 = call-poly <vilib>:"Write To Spreadsheet File.vi"("transpose? (no:F)"=TRUE, "format (%.3f)"=w467, "2D data"=w465, "file path (dialog if empty)"=w466) -> ()  [unwired: 4 in, 1 out]
                  n164 = call-poly <vilib>:"Write To Spreadsheet File.vi"("transpose? (no:F)"=TRUE, "format (%.3f)"=w467, "2D data"=w469, "file path (dialog if empty)"=w470) -> ("new file path (Not A Path if cancelled)"=w463:path)  [unwired: 4 in]
                }
                frame "WLC Fitting" {
                  n165 = call-poly <vilib>:"Write To Spreadsheet File.vi"("transpose? (no:F)"=TRUE, "format (%.3f)"="%.6f", "2D data"=w473, "file path (dialog if empty)"=w472) -> ("new file path (Not A Path if cancelled)"=w471:path)  [unwired: 4 in]
                }
              }
            }
          }
          "Save to Path" <- w447
        }
      }
    }
  }
